vi "Save Targets to Disc.vi"(0 "Internal Path":path, 1 "Internal Target Map":map{string, string}(c390), 2 "External Path":path, 3 "External Target Map":map{string, string}(c390), 4 "Unhandled Path":path, 5 "Unhandled Dependencies":string[](array[string]), 7 "error in (no error)":errorcluster) -> (27 "error out":errorcluster)   [LabVIEW 2019, in "Project.Dependencies Finder.lvlib" / "Dependency Source.lvclass"]
doc: "Save dependency source data to disc."
uses:
  Dependency Source.lvclass
  <vilib>/Utility/file.llb/Write Delimited Spreadsheet (string).vi
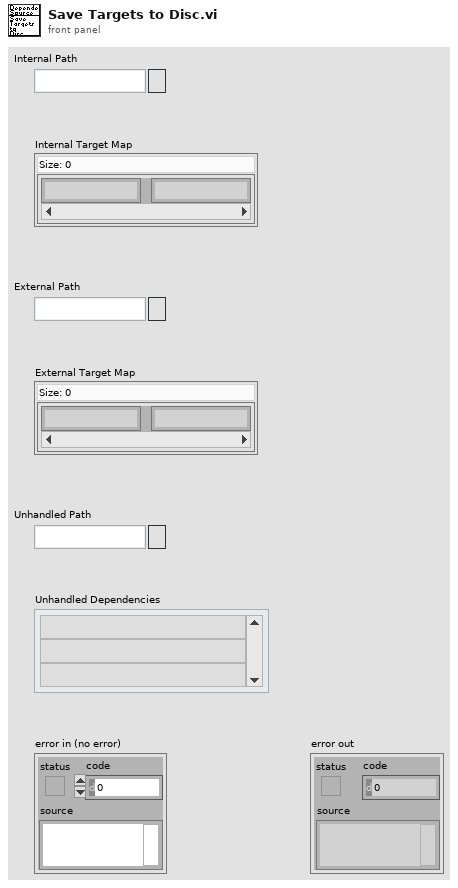
[diagram p1: front panel]
types:
  T1 = cluster{"Internal Path":path, "Internal Target Map":map{string, string}}
  T2 = cluster{"External Path":path, "External Target Map":map{string, string}}
  T3 = cluster{"External Path":path, "External Target Map":map{string, string}}[]
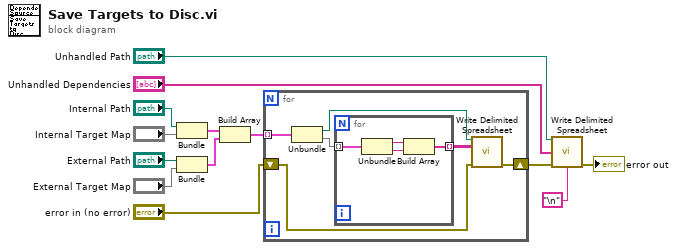
[diagram p0: block diagram]
diagram:
  n1 = Bundle("Internal Path"="Internal Path", "Internal Target Map"="Internal Target Map") -> (w9:T1)  [unwired: 1 in]
  n2 = Bundle("External Path"="External Path", "External Target Map"="External Target Map") -> (w8:T2)  [unwired: 1 in]
  n3 = Build Array(w9, w8) -> (w7:T3)
  n4 = for {
    tunnel: w7 -> [w19] mode=indexing
    shift-right: [w16] -> w5
    shift-left: "error in (no error)" -> [w17]
    n5 = Unbundle(w19) -> ("External Path"=w18:path, "External Target Map"=w15:map{string, string})
    n6 = for {
      tunnel: w15 -> [w23] mode=indexing
      tunnel: [w20] -> w14 mode=indexing
      n7 = Unbundle(w23) -> ("Unique Folder Name"=w22:string, "Dependency Name"=w21:string)
      n8 = Build Array(w22, w21) -> (w20:string[])
    }
    n9 = call-poly <vilib>:"Write Delimited Spreadsheet.vi"("file path (dialog if empty)"=w18, "2D data"=w14, "error in (no error)"=w17) -> ("error out"=w16:errorcluster)  [unwired: 11 in, 1 out]
  }
  n10 = call-poly <vilib>:"Write Delimited Spreadsheet.vi"("file path (dialog if empty)"="Unhandled Path", "1D data"="Unhandled Dependencies", "error in (no error)"=w5, "delimiter (\\t)"="\n") -> ("error out"=→"error out":errorcluster)  [unwired: 10 in, 1 out]
